vi "Amira Bladder Calibration - Multiple - V1.0.vi"() -> ()   [LabVIEW 2020]
uses:
  <userlib>/KQD LabVIEW User/Serial/Controls/SERIAL PortConfig.ctl
  <userlib>/KQD LabVIEW User/Serial/Controls/SERIAL BaudRate.ctl
  <userlib>/KQD LabVIEW User/Button/STOP.ctl
  <userlib>/Amira UART/Public/TypeDefs/AUART StepDir.ctl
  <userlib>/Amira UART/Amira UART.lvclass
  <userlib>/KQD LabVIEW User/Serial/Serial.lvlib
panel:
  in  "Stop":T1
  out "Idx":i32
  in  "Iteration":i32
  in  "RunWith":cluster{"Steps":i32, "Rates":i32}={"Steps"=400, "Rates"=40}
  in  "Folder":path=path "C:/Amira Data/Strip"
  in  "Strip":enum16{"Surface", "Blader"}(ring)
  out "FrontOpen":dbl
  out "BackOpen":dbl
  out "FrontClose":dbl
  out "BackClose":dbl
  in  "StartAt":cluster{"Steps":i32, "Rates":i32}={"Steps"=950, "Rates"=200}
  out "Position":dbl[](graph)
  in  "DAQ":tag="Dev1/port0"
  out "UART":string
  in  "ComPort":refnum<visa-resource-name>
  in  "Config":T2={"BaudRate"=enum."460800", "StopBits"=10, "DataBits"=8, "Parity"=enum."None", "FlowControl"=2, "TimeOut"=1000, "TermChar"=10, "ReadTermEn"=TRUE} {"TermChar" format="%.0x"; "FlowControl" items=["None", "XON/XOFF", "RTS/CTS", "XON/XOFF & RTS/CTS", "DTR/DSR", "XON/XOFF & DTR/DSR"]; "DataBits" min=5 max=8 step=1; "StopBits" items=["1.0"=10, "1.5"=15, "2.0"=20]}
  out "ErrOut":errorcluster
  in  "ErrIn":errorcluster
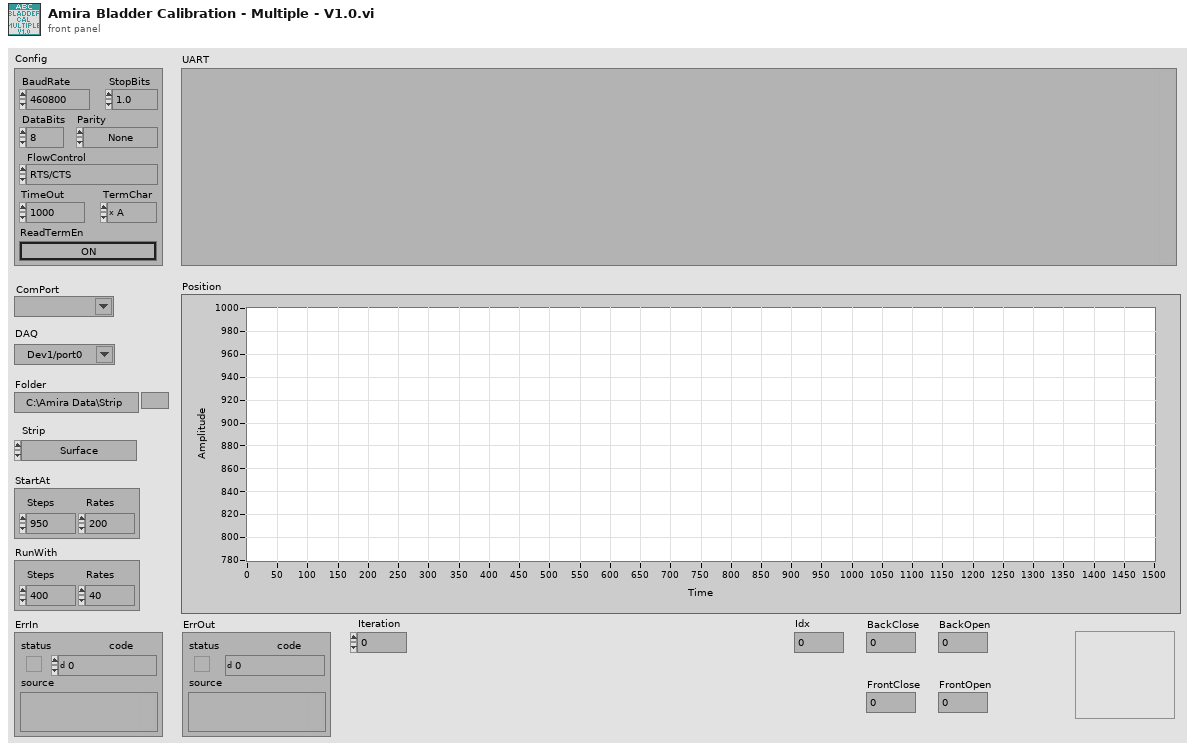
[diagram p1: front panel]
types:
  T1 = typedef "STOP.ctl" = bool
  T2 = typedef "Serial.lvlib/SERIAL PortConfig.ctl" = cluster{"BaudRate":T3, "StopBits":u16, "DataBits":u16, "Parity":enum16{"None", "Odd", "Even", "Mark", "Space"}, "FlowControl":u16, "TimeOut":u32, "TermChar":u8, "ReadTermEn":bool}
  T3 = typedef "SERIAL BaudRate.ctl" = enum16{"2400", "4800", "7200", "9600", "14400", "19200", "28800", "38400", "57600", "115200", "128000", "230400", "460800", "921600"}
  T4 = typedef "Amira UART.lvclass/AUART StepDir.ctl" = enum16{"", "compress", "decompress"}
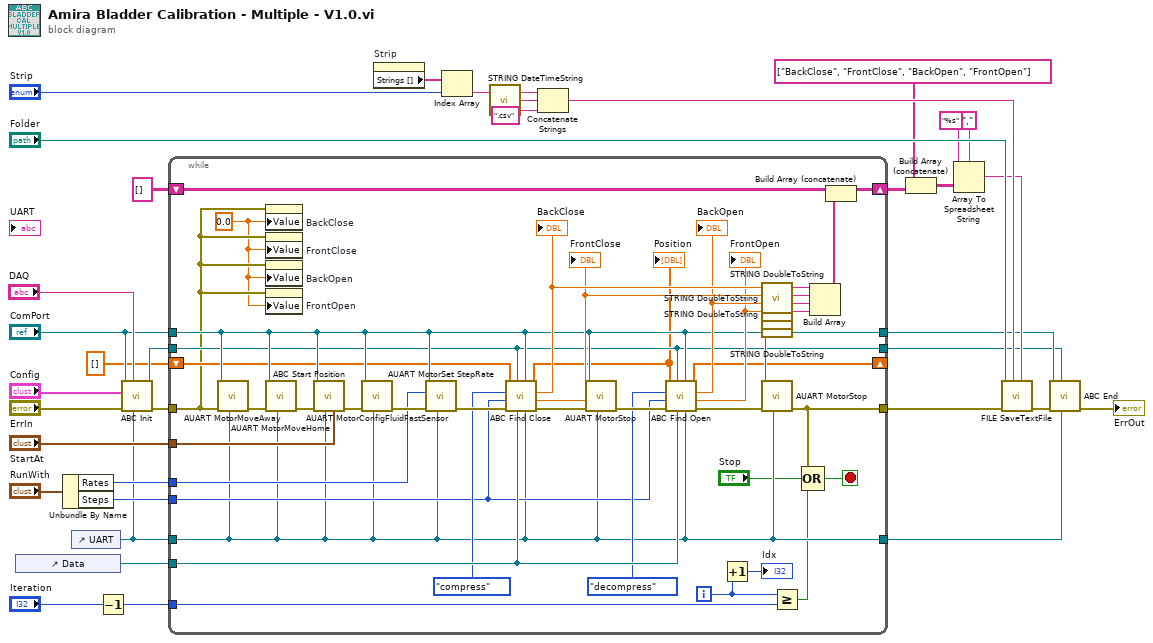
[diagram p0: block diagram]
diagram:
  n1 = control-ref of="Data"() -> (w30:refnum<vi>)
  n2 = Unbundle By Name("RunWith") -> ("Rates"=w16:i32, "Steps"=w15:i32)
  n3 = control-ref of="UART"() -> (w13:refnum<vi>)
  n4 = Decrement(x="Iteration") -> (x-1=w2:i32)
  n5 = call "ABC Init.vi"("UART"=w13, "DAQ"="DAQ", "ErrIn"="ErrIn", "PortConfig"="Config", "ComPort"="ComPort") -> ("ErrOut"=w14:errorcluster, "DaqTask"=w31:refnum<k21>)  [unwired: 5 in]
  n6 = while {
    tunnel: "StartAt" -> [w71]
    tunnel: w31 -> [w46]
    tunnel: w30 -> [w67]
    tunnel: w16 -> [w56]
    tunnel: w15 -> [w55]
    tunnel: w13 -> [w53]
    tunnel: "ComPort" -> [w47]
    tunnel: w14 -> [w40]
    tunnel: [w52] -> w11
    tunnel: [w53] -> w8
    tunnel: w2 -> [w50]
    tunnel: [w47] -> w6
    tunnel: [w46] -> w5
    shift-right: [w44] -> w3
    shift-left: string[][] [] -> [w43]
    shift-right: [w36] -> _
    shift-left: dbl[] [] ("DataOut") -> [w41]
    i -> [w51]
    stop <- w48 stop-if-true
    w39 = 0.0 ("BackClose")
    n7 = call <userlib>:"AUART MotorMoveAway.vi"("UART"=w53, "ErrIn"=w40, "Port"=w47) -> ("ErrOut"=w54:errorcluster)  [unwired: 8 in]
    n8 = property on="BackClose" class="DigNum (strict)"(error in=w40, "Value"=w39) -> ()  [unwired: 1 in, 2 out]
    n9 = property on="FrontClose" class="DigNum (strict)"(error in=w40, "Value"=w39) -> ()  [unwired: 1 in, 2 out]
    n10 = property on="BackOpen" class="DigNum (strict)"(error in=w40, "Value"=w39) -> ()  [unwired: 1 in, 2 out]
    n11 = property on="FrontOpen" class="DigNum (strict)"(error in=w40, "Value"=w39) -> ()  [unwired: 1 in, 2 out]
    n12 = call <userlib>:"AUART MotorMoveHome.vi"("UART"=w53, "ErrIn"=w54, "Port"=w47) -> ("ErrOut"=w73:errorcluster)  [unwired: 7 in, 1 out]
    n13 = call "ABC Start Position.vi"("Start"=w71, "UART"=w53, "ErrIn"=w73, "ComPort"=w47) -> ("ErrOut"=w72:errorcluster)  [unwired: 6 in, 1 out]
    n14 = call <userlib>:"AUART MotorConfigFluidFastSensor.vi"("UART"=w53, "ErrIn"=w72, "Port"=w47) -> ("ErrOut"=w75:errorcluster)  [unwired: 8 in]
    n15 = call <userlib>:"AUART MotorSet StepRate.vi"("UART"=w53, "ErrIn"=w75, "step_rate"=w56, "Port"=w47) -> ("ErrOut"=w74:errorcluster)  [unwired: 7 in]
    n16 = call "ABC Find Close.vi"("UART"=w53, "ComPort"=w47, "Data"=w67, "DaqTask"=w46, "ErrIn"=w74, "#Step"=w55, "Dir"=AUART_StepDir."compress" ("step_dir"), "DataIn"=w41) -> ("ErrOut"=w70:errorcluster, "FrontClose"=w65:dbl, "BackClose"=w66:dbl, "DataOut"=w42:dbl[])
    "Position" <- w42
    "BackClose" <- w66
    "FrontClose" <- w65
    n17 = call <userlib>:"AUART MotorStop.vi"("UART"=w53, "ErrIn"=w70, "Port"=w47) -> ("ErrOut"=w69:errorcluster)  [unwired: 8 in]
    n18 = call "ABC Find Open.vi"("UART"=w53, "ComPort"=w47, "Data"=w67, "DaqTask"=w46, "ErrIn"=w69, "#Step"=w55, "Dir"=AUART_StepDir."decompress" ("step_dir"), "DataIn"=w42) -> ("ErrOut"=w68:errorcluster, "FrontOpen"=w63:dbl, "BackOpen"=w64:dbl, "DataOut"=w36:dbl[])
    "BackOpen" <- w64
    "FrontOpen" <- w63
    n19 = Increment(x=w51) -> (x+1=→"Idx":i32)
    n20 = call <userlib>:"STRING DoubleToString.vi"("Num"=w66) -> ("DblStr"=w62:string)  [unwired: 3 in]
    n21 = call <userlib>:"STRING DoubleToString.vi"("Num"=w65) -> ("DblStr"=w61:string)  [unwired: 3 in]
    n22 = call <userlib>:"STRING DoubleToString.vi"("Num"=w64) -> ("DblStr"=w60:string)  [unwired: 3 in]
    n23 = call <userlib>:"STRING DoubleToString.vi"("Num"=w63) -> ("DblStr"=w59:string)  [unwired: 3 in]
    n24 = call <userlib>:"AUART MotorStop.vi"("UART"=w53, "ErrIn"=w68, "Port"=w47) -> ("ErrOut"=w52:errorcluster)  [unwired: 8 in]
    n25 = Greater Or Equal?(x=w51, y=w50) -> (x >= y?=w49:bool)
    n26 = Compound Arithmetic op=OR(w52, "Stop", w49) -> (w48:T1)
    n27 = Build Array(w62, w61, w60, w59) -> (w45:string[])
    n28 = Build Array (concatenate)(w43, w45) -> (w44:string[][])
  }
  n29 = property on="Strip" class="Enum (strict)"() -> ("Strings []"=w29:string[])  [unwired: 2 in, 2 out]
  n30 = Index Array(array=w29, index="Strip") -> (element=w27:string)
  n31 = call <userlib>:"STRING DateTimeString.vi"() -> ("DateTimeStr"=w26:string)  [unwired: 2 in]
  n32 = Concatenate Strings(w27, w26, ".csv" ("string")) -> (w23:string)
  n33 = Build Array (concatenate)(string[] ["BackClose", "FrontClose", "BackOpen", "FrontOpen"], w3) -> (w21:string[][])
  n34 = Array To Spreadsheet String(delimiter (Tab)=",", array=w21, 3:"%s" ("format string")) -> (spreadsheet string=w19:string)
  n35 = call <userlib>:"FILE SaveTextFile.vi"("Data"=w19, "File"=w23, "ErrIn"=w11, "Folder"="Folder") -> ("ErrOut"=w10:errorcluster)  [unwired: 7 in]
  n36 = call "ABC End.vi"("UART"=w8, "DaqTask"=w5, "ErrIn"=w10, "ComPort"=w6) -> ("ErrOut"=→"ErrOut":errorcluster)  [unwired: 7 in]
